vi "Set Select Device Event.vi"(8 "error in (no error)":errorcluster, 10 "Select Device":refnum<user-event>, 11 "DeviceListPanel in":refnum<class "DeviceListPanel.lvclass">) -> (0 "error out":errorcluster, 3 "DeviceListPanel out":refnum<class "DeviceListPanel.lvclass">)   [LabVIEW 2020, in "PicoG-App.lvlib" / "DeviceListPanel.lvclass"]
uses:
  DeviceListPanel.lvclass
  Device/Device.lvclass
  DeviceListPanel.lvclass/DeviceListPanel.ctl
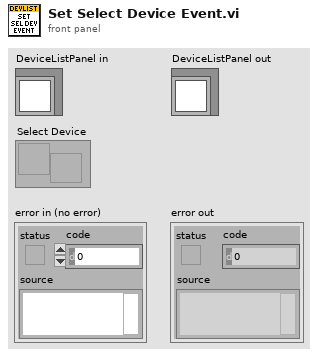
[diagram p1: front panel]
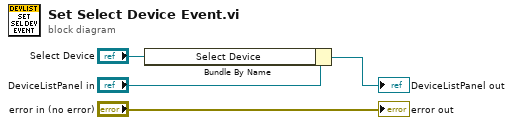
[diagram p0: block diagram]
diagram:
  n1 = Bundle By Name(cluster="DeviceListPanel in", "Select Device"="Select Device") -> (→"DeviceListPanel out":refnum<class "DeviceListPanel.lvclass">)
  "error out" <- "error in (no error)"
